vi "Start_Server_Cmd.vi"(8 "error in (no error)":errorcluster, 10 "command line":string="src/redis-server", 11 "working directory":path) -> (0 "error out":errorcluster, 2 "return code":i32)   [LabVIEW 2023]
panel:
  out "standard error":string
  out "standard output":string
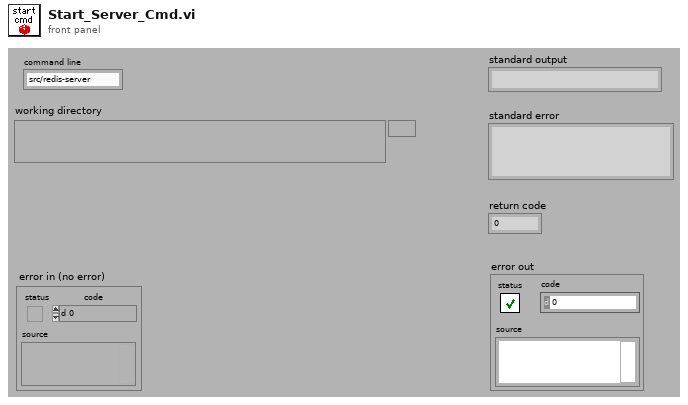
[diagram p1: front panel]
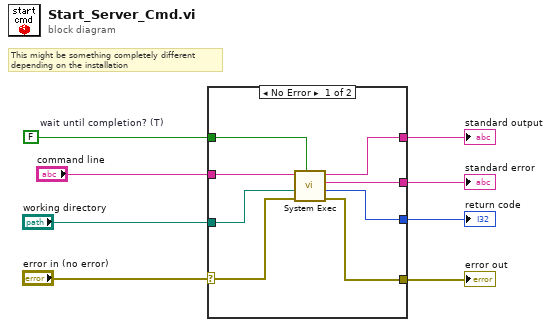
[diagram p0: block diagram]
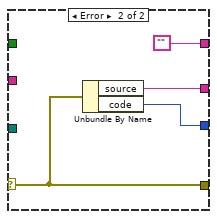
[diagram p2: hidden frame]
diagram:
  w8 = FALSE  # wait until completion? (T)
  # "This might be something completely different\ndepending on the installation"
  n1 = case shown="No Error" "error in (no error)" {
    selector: "error in (no error)" -> [w13 w20]
    tunnel: w8 -> [w16 _]
    tunnel: "command line" -> [w15 _]
    tunnel: "working directory" -> [w14 _]
    tunnel: [w12 "" ("standard output")] -> w4
    tunnel: [w11 w18] -> w3
    tunnel: [w10 w19] -> w2
    tunnel: [w9 w20] -> w1
    frame No Error {
      n2 = call <vilib>:"System Exec.vi"("wait until completion? (T)"=w16, "error in (no error)"=w13, "working directory"=w14, "command line"=w15) -> ("error out"=w9:errorcluster, "return code"=w10:i32, "standard error"=w11:string, "standard output"=w12:string)  [unwired: 4 in]
    }
    frame Error {
      n3 = Unbundle By Name(w20) -> ("source"=w18:string, "code"=w19:i32)
    }
  }
  "standard output" <- w4
  "standard error" <- w3
  "return code" <- w2
  "error out" <- w1
